vi "RunEmergencyStop86.vi"(4 "error in (no error)":errorcluster) -> ()   [LabVIEW 2010]
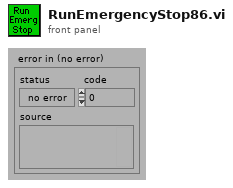
[diagram p1: front panel]
types:
  T1 = enum32{"Bad", "Idle", "Run top level", "Running"}
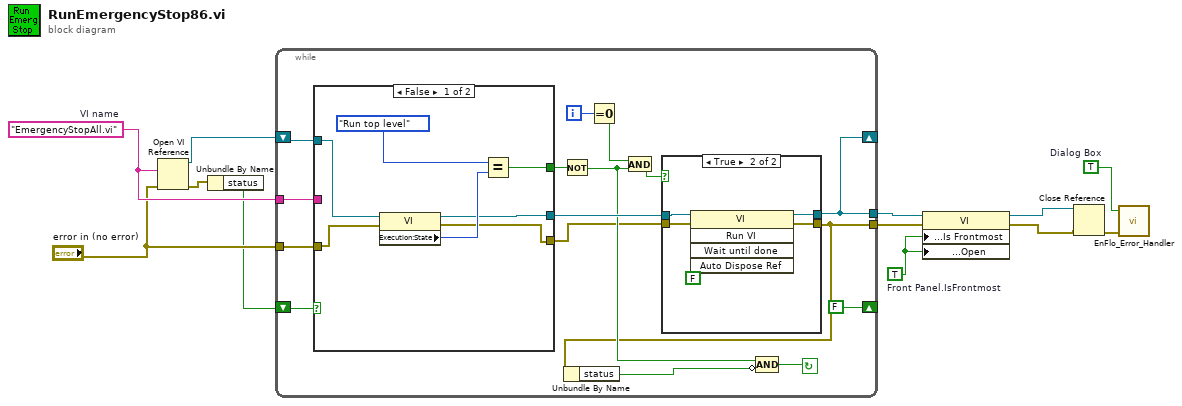
[diagram p0: block diagram]
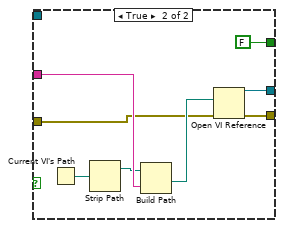
[diagram p3: hidden frame]
diagram:
  w4 = TRUE  # Dialog Box
  w1 = TRUE  # Front Panel.IsFrontmost
  w12 = "EmergencyStopAll.vi"  # VI name
  n1 = Open VI Reference(vi path=w12, error in (no error)="error in (no error)") -> (vi reference=w3:refnum<vi>, error out=w2:errorcluster)  [unwired: 1 in, 3 out]
  n2 = Unbundle By Name(w2) -> ("status"=w5:bool)
  n3 = while {
    shift-left: w3 -> [w16]
    shift-right: [w15] -> _
    shift-left: w5 -> [w25]
    shift-right: [FALSE] -> _
    tunnel: [w13] -> w8
    tunnel: [w15] -> w9
    tunnel: "error in (no error)" -> [w27]
    tunnel: w12 -> [w28]
    i -> [w22]
    stop <- w18 continue-if-true
    n4 = case shown="False" w25 {
      tunnel: w28 -> [_ w49]
      tunnel: w16 -> [w42 _]
      tunnel: w27 -> [w36 w46]
      tunnel: [w39 FALSE] -> w23
      tunnel: [w38 w45] -> w26
      tunnel: [w37 w44] -> w14
      frame False {
        n5 = property class="VI"(reference=w42, error in=w36) -> (reference out=w38:refnum<vi>, error out=w37:errorcluster, "Execution:State"=w41:T1)
        n6 = Equal?(x=T1."Run top level" ("Exec.State"), y=w41) -> (x = y?=w39:bool)
      }
      frame True {
        n7 = Current VI's Path() -> (path=w50:path)
        n8 = Strip Path(path=w50) -> (stripped path=w48:path)  [unwired: 1 out]
        n9 = Build Path(base path=w48, name or relative path=w49) -> (appended path=w47:path)
        n10 = Open VI Reference(vi path=w47, error in (no error)=w46) -> (vi reference=w45:refnum<vi>, error out=w44:errorcluster)  [unwired: 1 in, 3 out]
      }
    }
    n11 = Not(x=w23) -> (.not. x?=w17:bool)
    n12 = Equal To 0?(x=w22) -> (x = 0?=w21:bool)
    n13 = And(x=w21, y=w17) -> (x .and. y?=w20:bool)
    n14 = case shown="True" w20 {
      tunnel: w26 -> [w29 w33]
      tunnel: w14 -> [w30 w35]
      tunnel: [w30 w32] -> w13
      tunnel: [w29 w31] -> w15
      frame False {
      }
      frame True {
        n15 = invoke class="VI" method="Run VI"(reference=w33, error in=w35, "Wait until done"=FALSE) -> (reference out=w31:refnum<vi>, error out=w32:errorcluster)  [unwired: 2 in, 3 out]
      }
    }
    n16 = Unbundle By Name(w13) -> ("status"=w19:bool)
    n17 = Compound Arithmetic op=AND(w17, invert w19) -> (w18:bool)
  }
  n18 = property class="VI"(reference=w9, error in=w8, "Front Panel Window:Is Frontmost"=w1, "Front Panel Window:Open"=w1) -> (reference out=w6:refnum<vi>, error out=w7:errorcluster)
  n19 = Close Reference(reference=w6, error in (no error)=w7) -> (error out=w10:errorcluster)
  n20 = call "EnFlo_Error_Handler.vi"("error in (no error)"=w10, "Dialog Box (T)"=w4) -> ()  [unwired: 1 in, 3 out]
